vi "logForceActuatorInfo.vi"(8 "error in (no error)":errorcluster, 10 "EventForceActuatorInfo":T1, 11 "Communicator in":refnum<class "Communicator.lvclass">) -> (0 "error out":errorcluster, 3 "Communicator out":refnum<class "Communicator.lvclass">)   [LabVIEW 2016, in "M1M3SupportCommunicator.lvlib" / "Communicator.lvclass"]
uses:
  Communicator.lvclass
  DataTypes/Topics/EventForceActuatorInfo.ctl
  DataTypes/Topics/Parts/Timestamp.ctl
  DataTypes/Topics/M1M3SupportTopics.lvlib
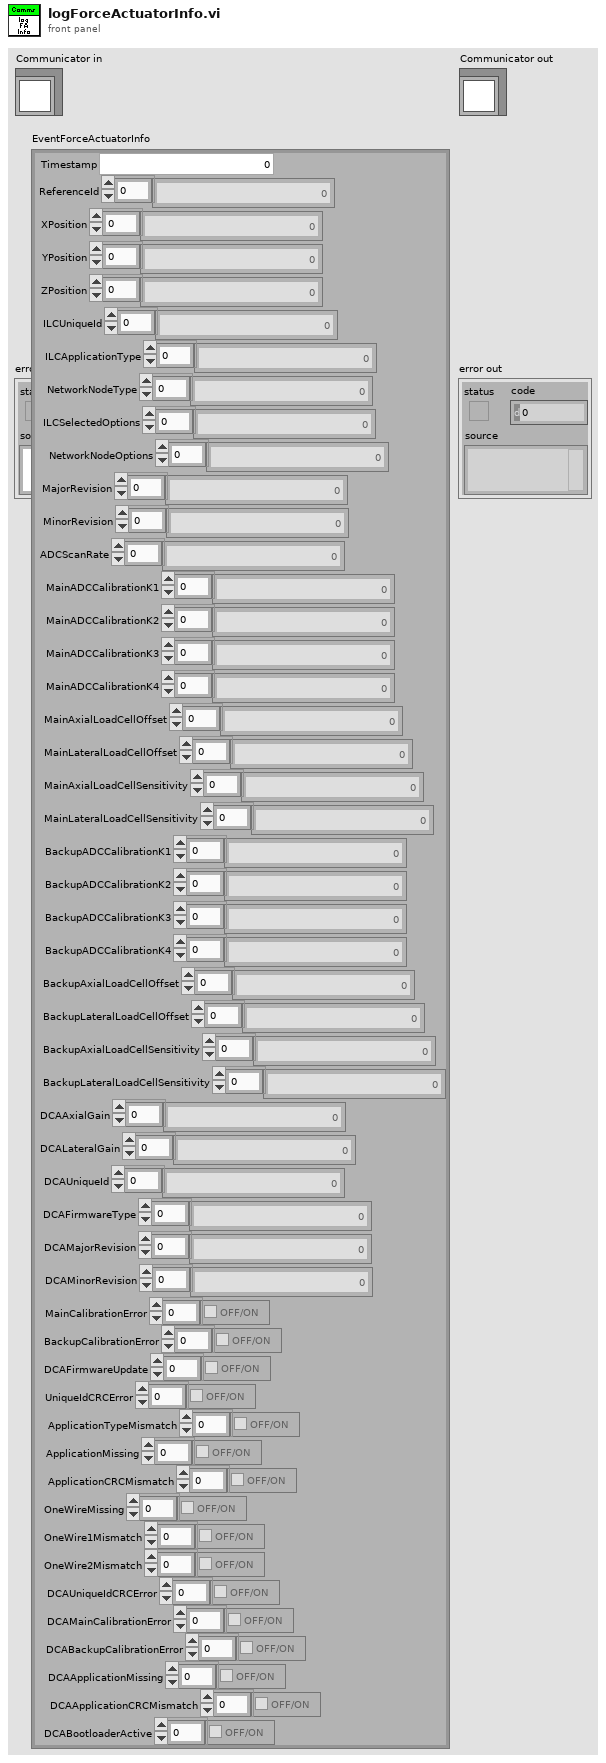
[diagram p1: front panel]
types:
  T1 = typedef "M1M3SupportTopics.lvlib/EventForceActuatorInfo.ctl" = cluster{"Timestamp":T2, "ReferenceId":i32[], "XPosition":sgl[], "YPosition":sgl[], "ZPosition":sgl[], "ILCUniqueId":i64[], "ILCApplicationType":u8[], "NetworkNodeType":u8[], "ILCSelectedOptions":u8[], "NetworkNodeOptions":u8[], "MajorRevision":u8[], "MinorRevision":u8[], "ADCScanRate":u8[], "MainADCCalibrationK1":sgl[], "MainADCCalibrationK2":sgl[], "MainADCCalibrationK3":sgl[], "MainADCCalibrationK4":sgl[], "MainAxialLoadCellOffset":sgl[], "MainLateralLoadCellOffset":sgl[], "MainAxialLoadCellSensitivity":sgl[], "MainLateralLoadCellSensitivity":sgl[], "BackupADCCalibrationK1":sgl[], "BackupADCCalibrationK2":sgl[], "BackupADCCalibrationK3":sgl[], "BackupADCCalibrationK4":sgl[], "BackupAxialLoadCellOffset":sgl[], "BackupLateralLoadCellOffset":sgl[], "BackupAxialLoadCellSensitivity":sgl[], "BackupLateralLoadCellSensitivity":sgl[], "DCAAxialGain":sgl[], "DCALateralGain":sgl[], "DCAUniqueId":i64[], "DCAFirmwareType":u8[], "DCAMajorRevision":u8[], "DCAMinorRevision":u8[], "MainCalibrationError":bool[], "BackupCalibrationError":bool[], "DCAFirmwareUpdate":bool[], "UniqueIdCRCError":bool[], "ApplicationTypeMismatch":bool[], "ApplicationMissing":bool[], "ApplicationCRCMismatch":bool[], "OneWireMissing":bool[], "OneWire1Mismatch":bool[], "OneWire2Mismatch":bool[], "DCAUniqueIdCRCError":bool[], "DCAMainCalibrationError":bool[], "DCABackupCalibrationError":bool[], "DCAApplicationMissing":bool[], "DCAApplicationCRCMismatch":bool[], "DCABootloaderActive":bool[]}
  T2 = typedef "M1M3SupportTopics.lvlib/Timestamp.ctl" = dbl
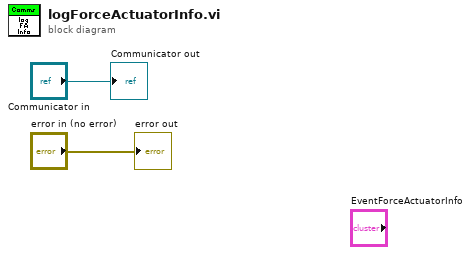
[diagram p0: block diagram]
diagram:
  "error out" <- "error in (no error)"
  "Communicator out" <- "Communicator in"
